vi "DropVI_ClientExampleCode.vi"() -> ()   [LabVIEW 2013, in "MQTT Client.lvlib"]
uses:
  MQTT Client.lvlib
  <vilib>/LabVIEW Open Source Project/Connection/Connection/Connection.lvclass
  Client class/Client.lvclass/Client.ctl
  <vilib>/LabVIEW Open Source Project/MQTT Connection/MQTT_Base/Base Class/MQTT_Base.lvclass/MQTT_Base.ctl
  <vilib>/LabVIEW Open Source Project/MQTT Control Packets/Control Packets/ControlPacket/ControlPacket.lvclass/ControlPacket.ctl
  <vilib>/LabVIEW Open Source Project/MQTT Control Packets/Control Packets/PUBLISH/PUBLISH.lvclass
  Client class/Client.lvclass
  <vilib>/LabVIEW Open Source Project/MQTT Connection/MQTT_Base/Base Class/MQTT_Base.lvclass
  <vilib>/LabVIEW Open Source Project/MQTT Control Packets/Control Packets/ControlPacket/ControlPacket.lvclass
panel:
  out "error out":errorcluster
  out "Published":bool
  out "Suback":bool
  out "Incoming Message":u8[](array[numeric]) format="%08b"
  in  "Subscribe":bool
  in  "Stop Client":bool
  in  "Publish":bool
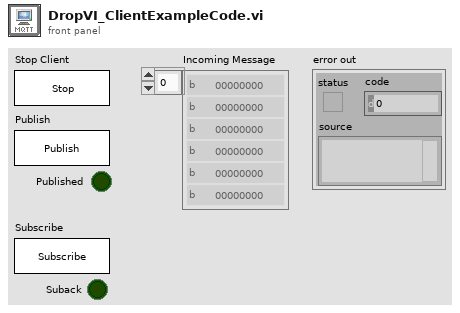
[diagram p1: front panel]
types:
  T1 = typedef "MQTT Client.lvlib/Client.lvclass/Public Events -- cluster.ctl" = cluster{"Connection Status":refnum<user-event>, "Connected":refnum<user-event>, "Application Message":refnum<user-event>}
  T2 = typedef "MQTT Base.lvlib/MQTT_Base.lvclass/Public Events -- cluster.ctl" = cluster{"Stop Event":refnum<user-event>, "Error Event":refnum<user-event>, "Inbound Message":refnum<user-event>}
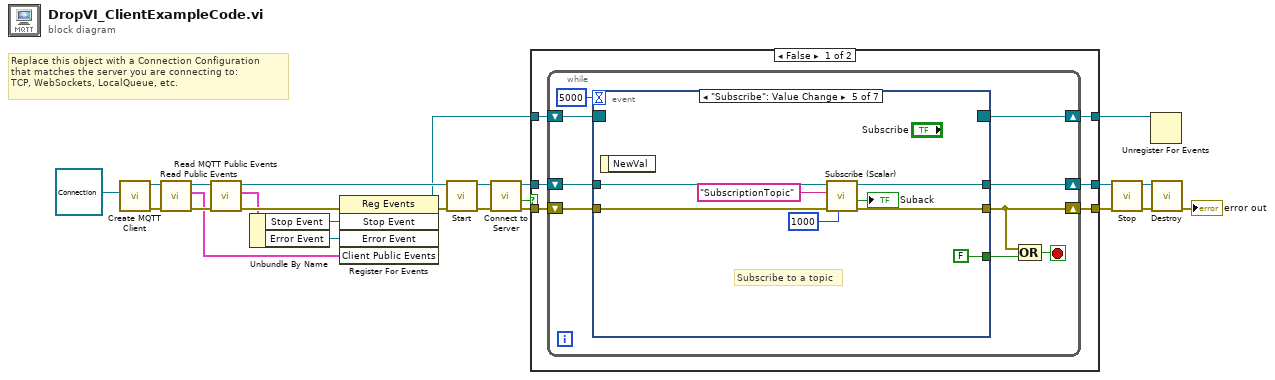
[diagram p0: block diagram]
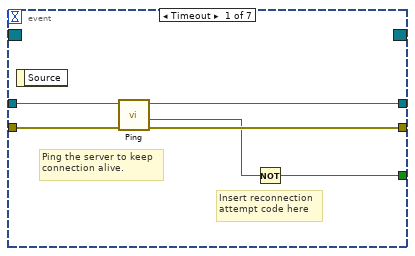
[diagram p2: hidden frame]
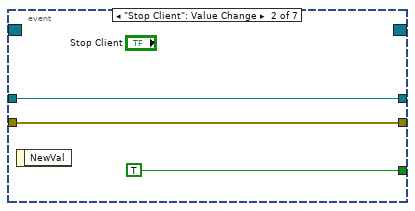
[diagram p3: hidden frame]
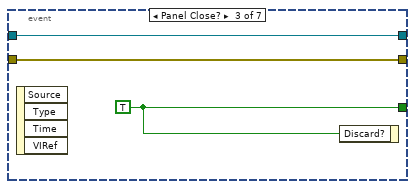
[diagram p4: hidden frame]
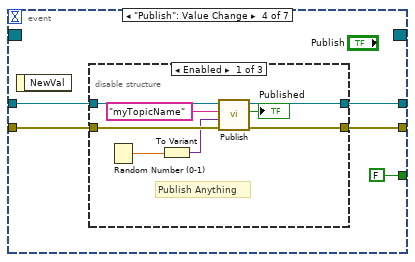
[diagram p5: hidden frame]
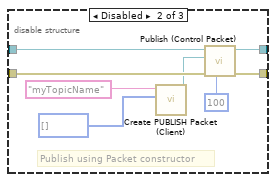
[diagram p6: hidden frame]
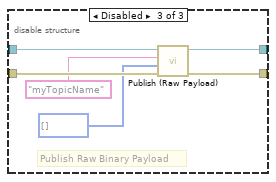
[diagram p7: hidden frame]
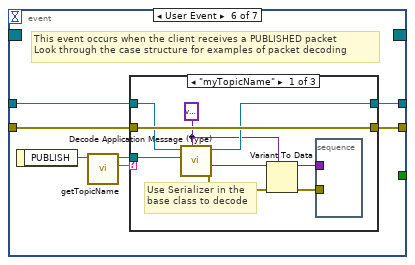
[diagram p8: hidden frame]
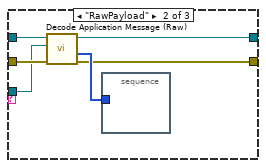
[diagram p9: hidden frame]
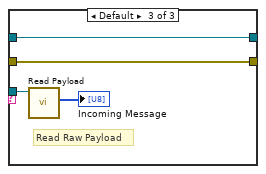
[diagram p10: hidden frame]
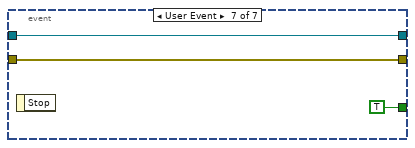
[diagram p11: hidden frame]
diagram:
  # "Replace this object with a Connection Configuration\nthat matches the server you are connecting to:\nTCP, WebSockets, LocalQueue, etc."
  n1 = call "Create MQTT Client.vi"("Connection Configuration"=refnum<class "Connection.lvclass"> refnum) -> ("error out"=w22:errorcluster, "Client out"=w24:refnum<class "Client.lvclass">)  [unwired: 9 in]
  n2 = call "Read Public Events.vi"("error in (no error)"=w22, "Client in"=w24) -> ("error out"=w21:errorcluster, "Client Public Events"=w19:T1, "Client out"=w23:refnum<class "Client.lvclass">)  [unwired: 7 in]
  n3 = call <vilib>:"Read MQTT Public Events.vi"("error in (no error)"=w21, "MQTT_Base in"=w23) -> ("error out"=w20:errorcluster, "MQTT Public Events"=w7:T2, "MQTT_Base out"=w17:refnum<class "Client.lvclass">)  [unwired: 7 in]
  n4 = Unbundle By Name(w7) -> ("Stop Event"=w9:refnum<user-event>, "Error Event"=w8:refnum<user-event>)
  n5 = register-events(error in=w20, w9, w8, w19) -> (reference out=w14:refnum<event-registration>, error out=w18:errorcluster)  [unwired: 1 in]
  n6 = call <vilib>:"Start.vi"("error in (no error)"=w18, "MQTT_Base in"=w17) -> ("error out"=w15:errorcluster, "MQTT_Base out"=w16:refnum<class "Client.lvclass">)  [unwired: 7 in, 1 out]
  n7 = call "Connect to Server.vi"("error in (no error)"=w15, "Client in"=w16) -> ("error out"=w11:errorcluster, "timed out"=w12:bool, "Client out"=w10:refnum<class "Client.lvclass">)  [unwired: 6 in, 1 out]
  n8 = case shown="False" w12 {
    tunnel: w14 -> [w30 w118]
    tunnel: [w29 w118] -> w13
    tunnel: w11 -> [w26 w116]
    tunnel: w10 -> [w28 w117]
    tunnel: [w27 w117] -> w5
    tunnel: [w25 w116] -> w3
    frame False {
      n9 = while {
        shift-right: [w38] -> w29
        shift-left: w30 -> [w39]
        shift-right: [w31] -> w27
        shift-left: w28 -> [w32]
        shift-right: [w36] -> w25
        shift-left: w26 -> [w37]
        stop <- w35 stop-if-true
        n10 = event shown="[4] \"Subscribe\": Value Change" {
          selector: w39 -> [_ _ _ _ _ _ _]
          dyn-events: [_ _ _ _ _ _ _] -> w38
          timeout: 5000 -> [_ _ _ _ _ _ _]
          tunnel: w37 -> [w44 w47 w49 w54 w83 w88 w115]
          tunnel: [w42 w47 w49 w53 w82 w89 w115] -> w36
          tunnel: [w41 TRUE w51 FALSE FALSE _ TRUE] -> w34
          tunnel: w32 -> [w45 w48 w50 w55 w85 w91 w113]
          tunnel: [w43 w48 w50 w52 w81 w90 w113] -> w31
          event Timeout {
            # "Insert reconnection\nattempt code here"
            # "Ping the server to keep\nconnection alive."
            n11 = event-data() -> ()  [unwired: 1 in, 1 out]
            n12 = call "Ping.vi"("error in (no error)"=w44, "Client in"=w45) -> ("error out"=w42:errorcluster, "Server responded"=w40:bool, "Client out"=w43:refnum<class "Client.lvclass">)  [unwired: 6 in, 1 out]
            n13 = Not(x=w40) -> (.not. x?=w41:bool)
          }
          event "Stop Client": Value Change {
            n14 = event-data() -> ()  [unwired: 1 in, 1 out]
          }
          event Panel Close? {
            w51 = TRUE
            n15 = event-data() -> ()  [unwired: 1 in, 4 out]
            n16 = event-data("Discard?"=w51) -> ()  [unwired: 1 in, 1 out]
          }
          event "Publish": Value Change {
            n17 = event-data() -> ()  [unwired: 1 in, 1 out]
            n18 = disable-structure shown="Enabled" {
              disable-tunnel: w55 -> [w64 w70 w78]
              disable-tunnel: w54 -> [w63 w68 w75]
              disable-tunnel: [w62 w67 w76] -> w53
              disable-tunnel: [w61 w69 w77] -> w52
              frame Enabled {
                # "Publish Anything"
                n19 = Random Number (0-1)() -> (number: 0 to 1=w59:dbl)
                n20 = To Variant(anything=w59) -> (Variant=w58:variant)
                n21 = call "Publish.vi"("error in (no error)"=w63, "Payload"=w58, "Topic Name (empty: Payload name)"="myTopicName", "Client in"=w64) -> ("error out"=w62:errorcluster, "Published"=→"Published":bool, "Client out"=w61:refnum<class "Client.lvclass">)  [unwired: 5 in]
              }
              frame Disabled {
                # "Publish using Packet constructor"
                n22 = call <vilib>:"Create PUBLISH Packet (Client).vi"("Payload"=u8[] [], "Topic Name"="myTopicName" ("Topic Name (empty: Payload name)")) -> ("PUBLISH"=w65:refnum<class "PUBLISH.lvclass">)  [unwired: 6 in, 3 out]
                n23 = call "Publish (Control Packet).vi"("timeout (1000ms)"=100 ("timeout (0ms : no ack)"), "error in (no error)"=w68, "PUBLISH"=w65, "Client in"=w70) -> ("error out"=w67:errorcluster, "Client out"=w69:refnum<class "Client.lvclass">)  [unwired: 5 in, 1 out]
              }
              frame Disabled {
                # "Publish Raw Binary Payload"
                n24 = call "Publish (Raw Payload).vi"("error in (no error)"=w75, "Binary Payload"=u8[] [] ("Payload"), "Topic Name"="myTopicName" ("Topic Name (empty: Payload name)"), "Client in"=w78) -> ("error out"=w76:errorcluster, "Client out"=w77:refnum<class "Client.lvclass">)  [unwired: 5 in, 1 out]
              }
            }
          }
          event "Subscribe": Value Change {
            # "Subscribe to a topic"
            n25 = event-data() -> ()  [unwired: 1 in, 1 out]
            n26 = call "Subscribe (Scalar).vi"("timeout (1000ms)"=1000 ("timeout (100ms)"), "error in (no error)"=w83, "Topic Filter"="SubscriptionTopic" ("Topic Name (empty: Payload name)"), "Client in"=w85) -> ("error out"=w82:errorcluster, "Ack"=→"Suback":bool, "Client out"=w81:refnum<class "Client.lvclass">)  [unwired: 5 in]
          }
          event User Event {
            # "This event occurs when the client receives a PUBLISHED packet\nLook through the case structure for examples of packet decoding"
            n27 = event-data() -> ("PUBLISH"=w93:refnum<class "PUBLISH.lvclass">)  [unwired: 1 in]
            n28 = call <vilib>:"getTopicName.vi"("PUBLISH in"=w93) -> ("Topic"=w92:string, "PUBLISH out"=w87:refnum<class "PUBLISH.lvclass">)  [unwired: 8 in, 1 out]
            n29 = case shown="\"myTopicName\"" w92 {
              tunnel: w91 -> [w99 w108 w112]
              tunnel: [w98 w107 w112] -> w90
              tunnel: [w102 w105 w111] -> w89
              tunnel: w88 -> [w102 w104 w111]
              tunnel: w87 -> [w97 w103 w110]
              frame "myTopicName" {
                w95 = variant ("Type")
                # "Use Serializer in the\nbase class to decode"
                n30 = call "Decode Application Message (Type).vi"("Type"=w95, "PUBLISH"=w97, "Client in"=w99) -> ("error out"=w94:errorcluster, "Payload"=w96:variant, "Client out"=w98:refnum<class "Client.lvclass">)  [unwired: 5 in, 1 out]
                n31 = Variant To Data(error in=w94, type=w95, Variant=w96) -> (data=w101:variant, error out=w100:errorcluster)
                n32 = stacked-sequence {
                  tunnel: w101 -> [_]
                  tunnel: w100 -> [_]
                  frame #0 {
                  }
                }
              }
              frame "RawPayload" {
                n33 = call "Decode Application Message (Raw).vi"("error in (no error)"=w104, "PUBLISH"=w103, "Client in"=w108) -> ("error out"=w105:errorcluster, "Payload"=w106:u8[], "Client out"=w107:refnum<class "Client.lvclass">)  [unwired: 5 in, 1 out]
                n34 = stacked-sequence {
                  tunnel: w106 -> [_]
                  frame #0 {
                  }
                }
              }
              frame Default {
                # "Read Raw Payload"
                n35 = call <vilib>:"Read Payload.vi"("ControlPacket in"=w110) -> ("Payload"=→"Incoming Message":u8[])  [unwired: 9 in, 1 out]
              }
            }
          }
          event User Event {
            n36 = event-data() -> ()  [unwired: 1 in, 1 out]
          }
        }
        n37 = Compound Arithmetic op=OR(w36, w34) -> (w35:bool)
      }
    }
    frame True {
    }
  }
  n38 = call <vilib>:"Stop.vi"("error in (no error)"=w3, "MQTT_Base in"=w5) -> ("error out"=w4:errorcluster, "MQTT_Base out"=w6:refnum<class "Client.lvclass">)  [unwired: 7 in, 1 out]
  n39 = Unregister For Events(event registration refnum=w13) -> ()  [unwired: 1 in, 1 out]
  n40 = call <vilib>:"Destroy.vi"("error in (no error)"=w4, "MQTT_Base in"=w6) -> ("error out"=→"error out":errorcluster)  [unwired: 8 in, 1 out]
